vi "update time.vi"(8 "error in (no error)":errorcluster, 11 "Contador in":refnum<class "Contador.lvclass">) -> (0 "error out":errorcluster, 3 "Contador out":refnum<class "Contador.lvclass">)   [LabVIEW 2020, in "Contador.lvlib" / "Contador.lvclass"]
uses:
  Contador.lvclass
  Contador.lvclass/Contador.ctl
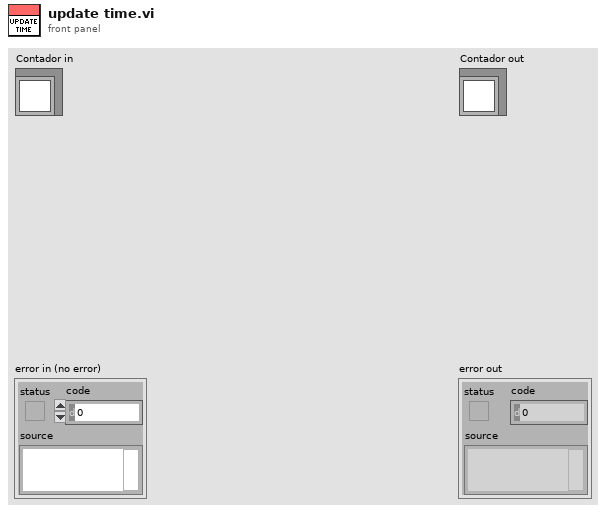
[diagram p1: front panel]
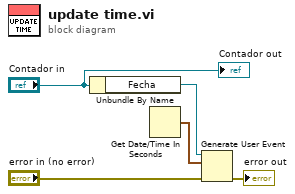
[diagram p0: block diagram]
diagram:
  n1 = Unbundle By Name("Contador in") -> ("Fecha"=w4:refnum<user-event>)
  n2 = Get Date/Time In Seconds() -> (seconds since 1Jan1904=w3:timestamp)
  n3 = Generate User Event(user event=w4, event data cluster=w3, error in="error in (no error)") -> (error out=→"error out":errorcluster)  [unwired: 1 in, 1 out]
  "Contador out" <- "Contador in"
